vi "CalcMean(String).vi"(0 "Array":string[][](array[string])) -> (1 "Red":dbl, 2 "Zero?":bool, 3 "Blue":dbl)   [LabVIEW 2013, in "main.lvlib"]
uses:
  main.lvlib
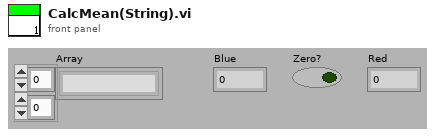
[diagram p1: front panel]
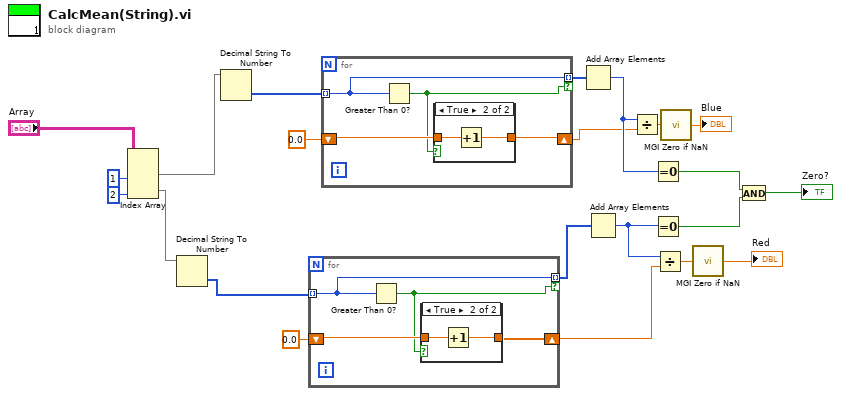
[diagram p0: block diagram]
diagram:
  n1 = Index Array(array="Array", index (col) #1=1 ("disabled index (col)"), index (col) #2=2 ("index (col)")) -> (element #1=w12:string[], element #2=w15:string[])  [unwired: 2 in]
  n2 = Decimal String To Number(string=w15) -> (number=w20:i32[])  [unwired: 2 in, 1 out]
  n3 = Decimal String To Number(string=w12) -> (number=w4:i32[])  [unwired: 2 in, 1 out]
  n4 = for {
    shift-right: [w26] -> w22
    shift-left: 0.0 -> [w25]
    tunnel: w20 -> [w24] mode=indexing
    tunnel: [w24] -> w6 mode=indexing if=w23
    n5 = Greater Than 0?(x=w24) -> (x > 0?=w23:bool)
    n6 = case shown="True" w23 {
      tunnel: [w27 w29] -> w26
      tunnel: w25 -> [w27 w28]
      frame False {
      }
      frame True {
        n7 = Increment(x=w28) -> (x+1=w29:dbl)
      }
    }
  }
  n8 = for {
    shift-right: [w33] -> w1
    shift-left: 0.0 -> [w32]
    tunnel: w4 -> [w31] mode=indexing
    tunnel: [w31] -> w3 mode=indexing if=w30
    n9 = Greater Than 0?(x=w31) -> (x > 0?=w30:bool)
    n10 = case shown="True" w30 {
      tunnel: [w34 w36] -> w33
      tunnel: w32 -> [w34 w35]
      frame False {
      }
      frame True {
        n11 = Increment(x=w35) -> (x+1=w36:dbl)
      }
    }
  }
  n12 = Add Array Elements(numeric array=w3) -> (sum=w2:i32)
  n13 = Add Array Elements(numeric array=w6) -> (sum=w19:i32)
  n14 = Divide(x=w2, y=w1) -> (x/y=w8:dbl)
  n15 = Equal To 0?(x=w2) -> (x = 0?=w18:bool)
  n16 = Equal To 0?(x=w19) -> (x = 0?=w17:bool)
  n17 = Divide(x=w19, y=w22) -> (x/y=w10:dbl)
  n18 = call <userlib>:"MGI Zero if NaN.vi"("Number In"=w8) -> ("Number Out"=→"Blue":dbl)
  n19 = call <userlib>:"MGI Zero if NaN.vi"("Number In"=w10) -> ("Number Out"=→"Red":dbl)
  n20 = And(x=w18, y=w17) -> (x .and. y?=→"Zero?":bool)
